vi "Enumerate Services.vi"(7 "error in":errorcluster, 10 "request data":T4) -> (0 "error out":errorcluster, 3 "response data":T1)   [LabVIEW 2021, in "NI Discovery V1 Client.lvlib"]
uses:
  NI Discovery V1 Client.lvlib
  gRPC/Generated APIs/ni/measurementlink/discovery/v1/RPC Messages/ni_measurementlink_discovery_v1_EnumerateServicesRequest.ctl
  gRPC/Generated APIs/ni/measurementlink/discovery/v1/RPC Messages/ni_measurementlink_discovery_v1_EnumerateServicesResponse.ctl
  gRPC/Generated APIs/ni/measurementlink/discovery/v1/RPC Messages/ni_measurementlink_discovery_v1_ServiceDescriptor.ctl
  gRPC/Generated APIs/ni/measurementlink/discovery/v1/RPC Messages/ni_measurementlink_discovery_v1_ServiceDescriptor_AnnotationsEntry.ctl
  TypeDefs/gRPC Client Cache FGV Action.ctl
  gRPC/Generated APIs/ni/measurementlink/discovery/v1/ni.measurementlink.discovery.v1.api.lvlib
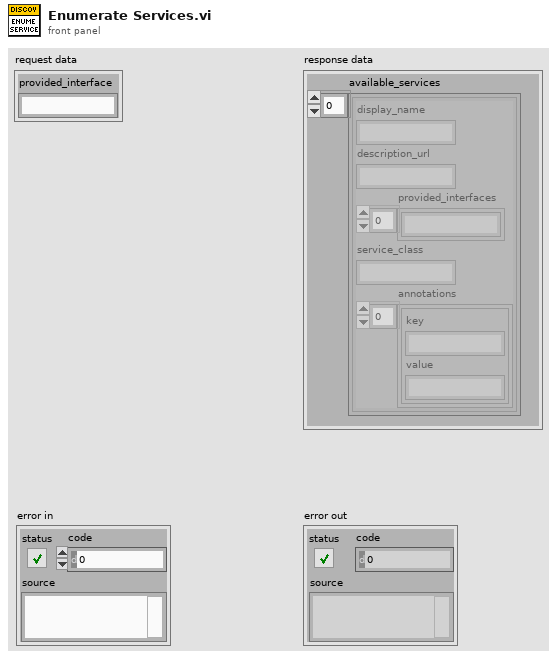
[diagram p1: front panel]
types:
  T1 = typedef "ni.measurementlink.discovery.v1.api.lvlib/ni_measurementlink_discovery_v1_EnumerateServicesResponse.ctl" = cluster{"available_services":T2[]}
  T2 = typedef "ni.measurementlink.discovery.v1.api.lvlib/ni_measurementlink_discovery_v1_ServiceDescriptor.ctl" = cluster{"display_name":string, "description_url":string, "provided_interfaces":string[], "service_class":string, "annotations":T3[]}
  T3 = typedef "ni.measurementlink.discovery.v1.api.lvlib/ni_measurementlink_discovery_v1_ServiceDescriptor_AnnotationsEntry.ctl" = cluster{"key":string, "value":string}
  T4 = typedef "ni.measurementlink.discovery.v1.api.lvlib/ni_measurementlink_discovery_v1_EnumerateServicesRequest.ctl" = cluster{"provided_interface":string}
  T5 = typedef "NI Discovery V1 Client.lvlib/gRPC Client Cache FGV Action.ctl" = enum16{"Get Client", "Recreate Client", "Destroy Client", "Update ClusterId"}
  T6 = typedef "grpc-lvsupport-release.lvlib/grpcId.ctl" = u64
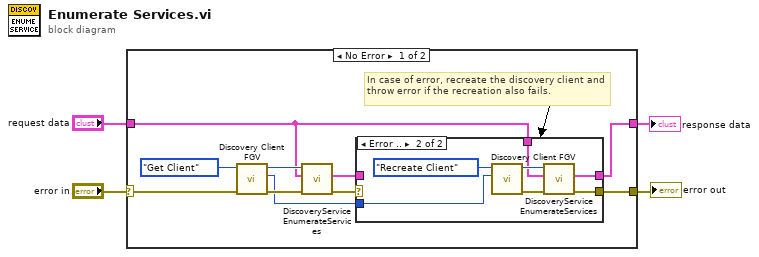
[diagram p0: block diagram]
diagram:
  n1 = case shown="No Error" "error in" {
    selector: "error in" -> [w14 w24]
    tunnel: [w9 w24] -> w1
    tunnel: [w8 _] -> w3
    tunnel: "request data" -> [w6 _]
    frame No Error {
      # "In case of error, recreate the discovery client and throw error if the recreation also fails."
      n2 = call "Discovery Client FGV.vi"("error in"=w14, "action"=gRPC_Client_Cache_FGV_Action."Get Client") -> ("error out"=w12:errorcluster, "unique id out"=w5:u64, "grpc client id"=w11:T6)  [unwired: 6 in, 1 out]
      n3 = call "DiscoveryService EnumerateServices.vi"("error in"=w12, "Request Data"=w6, "gRPC ID"=w11) -> ("error out"=w10:errorcluster, "Response Data"=w7:T1)  [unwired: 6 in, 1 out]
      n4 = case shown="Error .." w10 {
        selector: w10 -> [w16 _]
        tunnel: [w16 w20] -> w9
        tunnel: [w15 w17] -> w8
        tunnel: w7 -> [w15 _]
        tunnel: w6 -> [_ w19]
        tunnel: w5 -> [_ w18]
        frame No Error {
        }
        frame Error {
          n5 = call "Discovery Client FGV.vi"("unique id in"=w18, "action"=gRPC_Client_Cache_FGV_Action."Recreate Client") -> ("error out"=w21:errorcluster, "grpc client id"=w22:T6)  [unwired: 6 in, 2 out]
          n6 = call "DiscoveryService EnumerateServices.vi"("error in"=w21, "Request Data"=w19, "gRPC ID"=w22) -> ("error out"=w20:errorcluster, "Response Data"=w17:T1)  [unwired: 6 in, 1 out]
        }
      }
    }
    frame Error {
    }
  }
  "response data" <- w3
  "error out" <- w1
